vi "FindAvailableIDs.vi"(1 "All ids":i32[](array[numeric]), 2 "Unavailable ids":i32[](array[numeric])) -> (0 "available map id":i32[](array[numeric]))   [LabVIEW 2017, in "GetSetShared.lvlib"]
uses:
  <vilib>/express/express signal manip/GetorSetDDTAttributes/Shared VIs/GetSetShared.lvlib
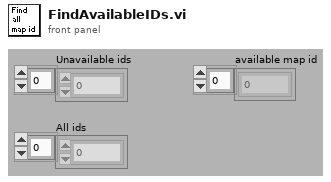
[diagram p1: front panel]
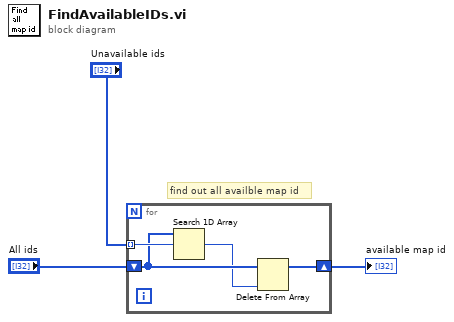
[diagram p0: block diagram]
diagram:
  # "find out all availble map id"
  n1 = for {
    tunnel: "Unavailable ids" -> [w7] mode=indexing
    shift-right: [w4] -> w2
    shift-left: "All ids" -> [w6]
    n2 = Search 1D Array(1D array=w6, element=w7) -> (index of element=w5:i32)  [unwired: 1 out]
    n3 = Delete From Array(array=w6, index=w5) -> (array with subset deleted=w4:i32[])  [unwired: 1 in, 1 out]
  }
  "available map id" <- w2
